vi "FTW-Message-Actor-Construct.vi"(8 "error in":errorcluster, 10 "Payload":variant, 11 "Parameter":string) -> (0 "error out":errorcluster, 3 "Actor Message":refnum<class "FTW-Message-Actor.lvclass">)   [LabVIEW 2013, in "FTW-Message-Actor.lvclass"]
uses:
  FTW-Message-Actor.lvclass
  FTW-Message-Actor.lvclass/FTW-Message-Actor.ctl
  Message/FTW-Message.lvclass
panel:
  # "Inputs"
  # "Outputs"
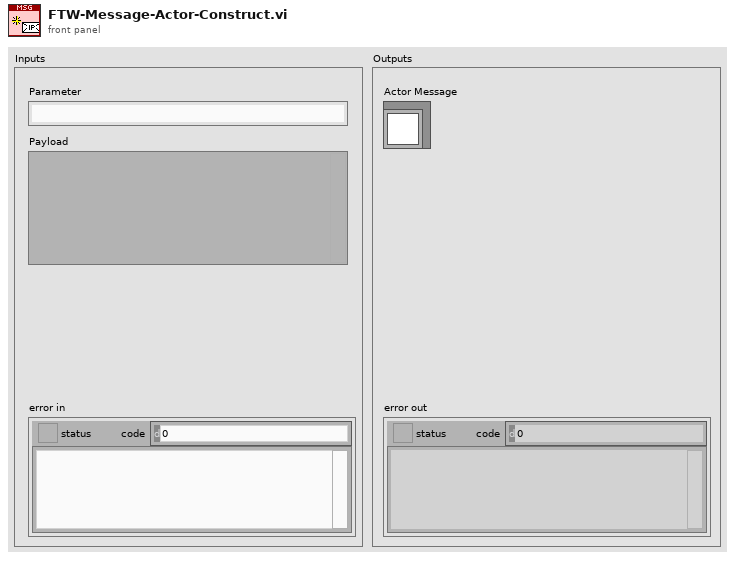
[diagram p1: front panel]
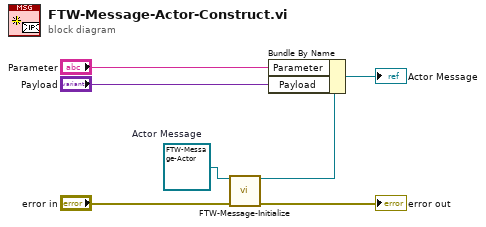
[diagram p0: block diagram]
diagram:
  w2 = refnum<class "FTW-Message-Actor.lvclass"> refnum  # Actor Message
  n1 = call "FTW-Message-Initialize.vi"("Message"=w2, "error in"="error in") -> ("Message out"=w3:refnum<class "FTW-Message-Actor.lvclass">, "error out"=→"error out":errorcluster)  [unwired: 12 in]
  n2 = Bundle By Name(cluster=w3, "Parameter"="Parameter", "Payload"="Payload") -> (→"Actor Message":refnum<class "FTW-Message-Actor.lvclass">)
